vi "Initialise.vi"(8 "error in (no error)":errorcluster, 11 "Node in":refnum<class "bt_WaitOn_Notifier.lvclass">) -> (0 "error out":errorcluster, 3 "Node out":refnum<class "bt_WaitOn_Notifier.lvclass">)   [LabVIEW 2021, in "BT.lvlib" / "bt_WaitOn_Notifier.lvclass"]
uses:
  bt_WaitOn_Notifier.lvclass
  bt_WaitOn_Notifier.lvclass/bt_WaitOn_Notifier.ctl
  Blackboard/Blackboard.lvclass/Blackboard.ctl
  <vilib>/TSA/Omni-Bus/Local Bus/Support/Initialise DVR's.vi
  <vilib>/TSA/Abstract Data Classes/Abs_Types/Value/Abs_Value.lvclass
  <vilib>/TSA/Abstract Data Classes/Abs_Types/Type/Abs_Type.lvclass
  With Values/WaitOn/bt_WaitOn_Synch_WithValues.lvclass
  Blackboard/Blackboard.lvclass
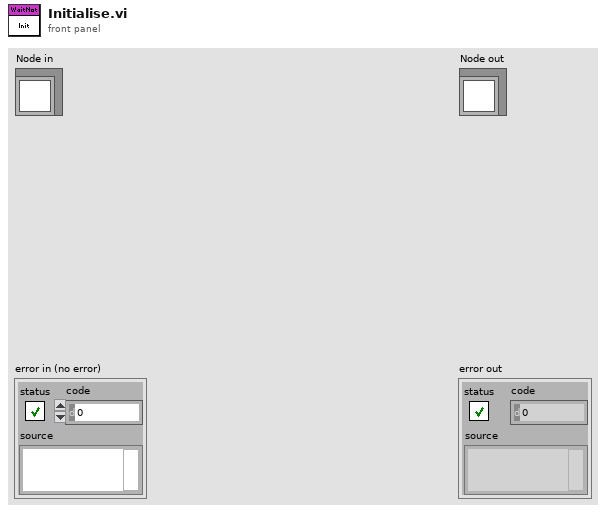
[diagram p1: front panel]
types:
  T1 = typedef "NI_Data Type.lvlib/Data Type.ctl" = enum8{"Invalid Type", "Void", "I8", "I16", "I32", "I64", "U8", "U16", "U32", "U64", "Single Float", "Double Float", "Extended Float", "Single Complex", "Double Complex", "Extended Complex", "Enum U8", "Enum U16", "Enum U32", "Enum U64", "Single Float With Unit", "Double Float With Unit", "Extended Float With Unit", "Single Complex with Unit", "Double Complex with Unit", "Extended Complex with Unit", "Boolean", "String", "Path", "Picture", "Tag", "Array", "Cluster", "Variant", "LV Variant", "Waveform", "Timestamp", "Digital Waveform", "Digital Data", "ExpressData", "Refnum", "External Data", "VI", "Poly VI", "LabVIEW Class Instance", "Fixed Point", "Set Collection", "Map Collection"}
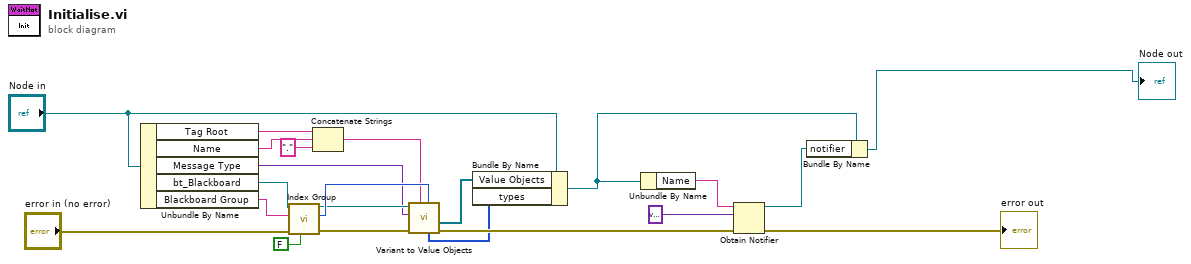
[diagram p0: block diagram]
diagram:
  n1 = Unbundle By Name("Node in") -> ("Tag Root"=w4:string, "Name"=w3:string, "Message Type"=w5:variant, "bt_Blackboard"=w7:refnum<class "Blackboard.lvclass">, "Blackboard Group"=w6:string)
  n2 = call "Index Group.vi"("Don't Create"=FALSE, "error in (no error)"="error in (no error)", "Group"=w6, "bt_Blackboard in"=w7) -> ("error out"=w14:errorcluster, "Index"=w16:i32, "bt_Blackboard out"=w15:refnum<class "Blackboard.lvclass">)  [unwired: 5 in]
  n3 = Concatenate Strings(w4, w3, "." ("string")) -> (w1:string)
  n4 = call "Variant to Value Objects.vi"("Group Index"=w16, "Name Root"=w1, "error in (no error)"=w14, "Variant"=w5, "bt_Blackboard in"=w15) -> ("error out"=w13:errorcluster, "Value Objects OUT"=w10:refnum<class "Abs_Value.lvclass">[], "types out"=w12:T1[])  [unwired: 3 in, 1 out]
  n5 = Bundle By Name(cluster="Node in", "Value Objects"=w10, "types"=w12) -> (w11:refnum<class "bt_WaitOn_Notifier.lvclass">)
  n6 = Unbundle By Name(w11) -> ("Name"=w20:string)
  n7 = Obtain Notifier(name (unnamed)=w20, notification data type=variant, error in (no error)=w13) -> (notifier out=w21:refnum<notifier>, error out=→"error out":errorcluster)  [unwired: 1 in, 1 out]
  n8 = Bundle By Name(cluster=w11, "notifier"=w21) -> (→"Node out":refnum<class "bt_WaitOn_Notifier.lvclass">)
